vi "Edge Counter.vi"(7 "Counter Parameters":T1={"Edge"=enum."Rising Edge", "Gate?"=FALSE, "Count Direction"=enum."Count Up", "Terminal Count"=16777216, "Ticks to Filter"=2, "High Pulse Time (us)"=1000}, 9 "Reset Counter":bool, 10 "Gate Input":bool, 11 "Ctr Source":bool) -> (1 "Terminal Count?":bool, 3 "Counter Register":u64)   [LabVIEW 2010]
doc: "This VI performs edge counting on the rising or falling edge of a digital signal source. It can also gate the signal and count in the up/down direction. It also determines when the terminal count is reached and output the counter register value."
uses:
  <userlib>/_NI VeriStand FPGA Support/NI VeriStand RIO Library/IP Based IO/Counter/common/CounterControl.ctl
panel:
  out "Filter Counter":u32
  out "Previous Ctr Source":bool
  out "Output Filtered Signal":bool
  # "ON"
  # "OFF"
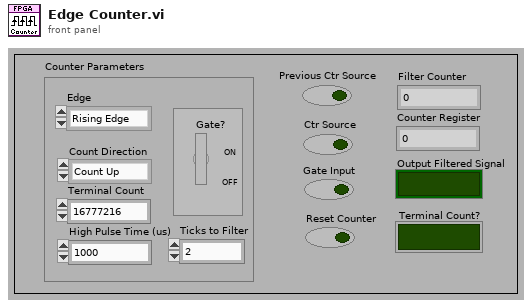
[diagram p1: front panel]
types:
  T1 = typedef "CounterControl.ctl" = cluster{"Edge":enum16{"Falling Edge", "Rising Edge"}, "Gate?":bool, "Count Direction":enum16{"Count Up", "Count Down"}, "Terminal Count":u64, "Ticks to Filter":u32, "High Pulse Time (us)":u32}
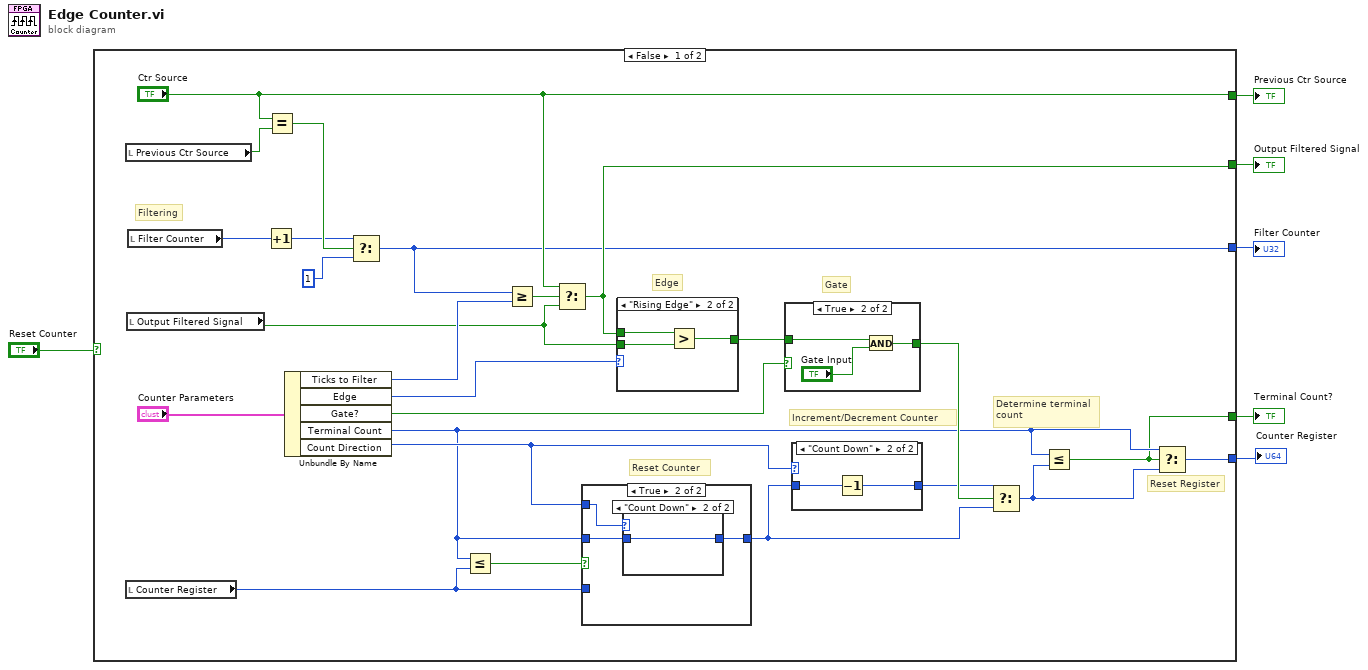
[diagram p0: block diagram]
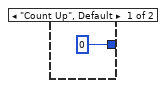
[diagram p3: hidden frame]
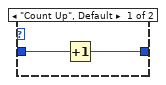
[diagram p4: hidden frame]
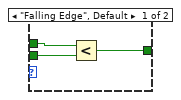
[diagram p6: hidden frame]
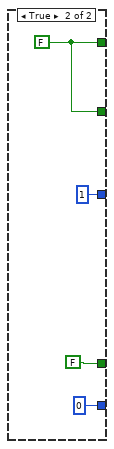
[diagram p7: hidden frame]
diagram:
  n1 = case shown="False" "Reset Counter" {
    tunnel: [w11 FALSE] -> w5
    tunnel: [w10 w55] -> w4
    tunnel: ["Ctr Source" w55] -> w3
    tunnel: [w8 u32 1 ("f")] -> w2
    tunnel: [w7 u64 0 ("Terminal Count")] -> w1
    frame False {
      # "Reset Register"
      # "Filtering"
      # "Determine terminal\ncount"
      # "Increment/Decrement Counter"
      # "Reset Counter"
      # "Edge"
      # "Gate"
      n2 = local read "Previous Ctr Source"() -> (w16:bool)
      n3 = local read "Counter Register"() -> (w14:u64)
      n4 = local read "Output Filtered Signal"() -> (w15:bool)
      n5 = local read "Filter Counter"() -> (w17:u32)
      n6 = Increment(x=w17) -> (x+1=w28:u32)
      n7 = Equal?(x="Ctr Source", y=w16) -> (x = y?=w29:bool)
      n8 = Unbundle By Name("Counter Parameters") -> ("Ticks to Filter"=w22:u32, "Edge"=w24:enum16{"Falling Edge", "Rising Edge"}, "Gate?"=w23:bool, "Terminal Count"=w13:u64, "Count Direction"=w21:enum16{"Count Up", "Count Down"})
      n9 = Select(t=w28, s=w29, f=u32 1) -> (s? t:f=w8:u32)
      n10 = Less Or Equal?(x=w13, y=w14) -> (x <= y?=w18:bool)
      n11 = Greater Or Equal?(x=w8, y=w22) -> (x >= y?=w26:bool)
      n12 = Select(t="Ctr Source", s=w26, f=w15) -> (s? t:f=w10:bool)
      n13 = case shown="True" w18 {
        tunnel: [w32 w34] -> w20
        tunnel: w14 -> [w32 _]
        tunnel: w13 -> [_ w33]
        tunnel: w21 -> [_ w35]
        frame False {
        }
        frame True {
          n14 = case shown="\"Count Down\"" w35 {
            tunnel: [u64 0 ("Register") w37] -> w34
            tunnel: w33 -> [_ w37]
            frame "Count Up", Default {
            }
            frame "Count Down" {
            }
          }
        }
      }
      n15 = case shown="\"Rising Edge\"" w24 {
        tunnel: w15 -> [w48 w50]
        tunnel: [w47 w51] -> w30
        tunnel: w10 -> [w46 w49]
        frame "Falling Edge", Default {
          n16 = Less?(x=w46, y=w48) -> (x < y?=w47:bool)
        }
        frame "Rising Edge" {
          n17 = Greater?(x=w49, y=w50) -> (0:w51:bool)
        }
      }
      n18 = case shown="True" w23 {
        tunnel: [w42 w45] -> w31
        tunnel: w30 -> [w42 w44]
        frame False {
        }
        frame True {
          n19 = And(x=w44, y="Gate Input") -> (x .and. y?=w45:bool)
        }
      }
      n20 = case shown="\"Count Down\"" w21 {
        tunnel: w20 -> [w39 w41]
        tunnel: [w38 w40] -> w19
        frame "Count Up", Default {
          n21 = Increment(x=w39) -> (x+1=w38:u64)
        }
        frame "Count Down" {
          n22 = Decrement(x=w41) -> (x-1=w40:u64)
        }
      }
      n23 = Select(t=w19, s=w31, f=w20) -> (s? t:f=w12:u64)
      n24 = Less Or Equal?(x=w13, y=w12) -> (x <= y?=w11:bool)
      n25 = Select(t=w13, s=w11, f=w12) -> (s? t:f=w7:u64)
    }
    frame True {
      w55 = FALSE ("Ctr Source")
    }
  }
  "Terminal Count?" <- w5
  "Output Filtered Signal" <- w4
  "Previous Ctr Source" <- w3
  "Filter Counter" <- w2
  "Counter Register" <- w1
